vi "getEnviada.vi"(11 "Cliente in":refnum<class "Cliente.lvclass">) -> (2 "msg_enviada":string, 3 "Cliente out":refnum<class "Cliente.lvclass">)   [LabVIEW 2015, in "Cliente.lvclass"]
uses:
  Cliente.lvclass
  Cliente.lvclass/Cliente.ctl
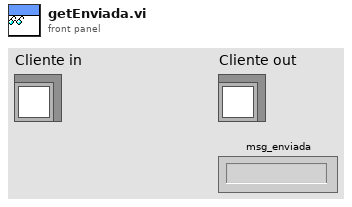
[diagram p1: front panel]
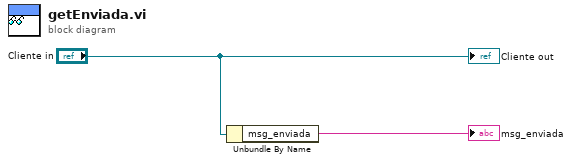
[diagram p0: block diagram]
diagram:
  n1 = Unbundle By Name("Cliente in") -> ("msg_enviada"=→"msg_enviada":string)
  "Cliente out" <- "Cliente in"
